vi "Enable Transient Operation.vi"(8 "error in (no error)":errorcluster, 10 "Enable Transient (T: Enable)":bool=TRUE, 11 "VISA resource name":refnum<visa-resource-name>) -> (0 "error out":errorcluster, 3 "VISA resource name out":refnum<visa-resource-name>)   [LabVIEW 2018, in "BK Precision 8600 Series.lvlib"]
doc: "Enable or disable the state of transient operation. Transient operation must be enabled first before sending a trigger to initiate the operation.\n\nRun this vi after configuring transient operation parameters using <b>Configure Transient Operation.vi</b>."
uses:
  <instrlib>/BK Precision 8600 Series/BK Precision 8600 Series.lvlib
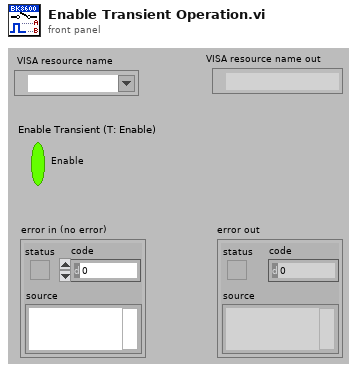
[diagram p1: front panel]
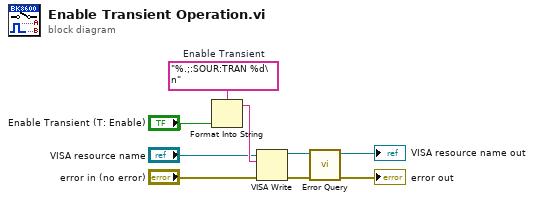
[diagram p0: block diagram]
diagram:
  w7 = "%.;:SOUR:TRAN %d\n"  # Enable Transient
  n1 = Format Into String(format string=w7, "Enable Transient (T: Enable)") -> (resulting string=w4:string)  [unwired: 2 in, 1 out]
  n2 = VISA Write(VISA resource name="VISA resource name", write buffer=w4, error in (no error)="error in (no error)") -> (VISA resource name out=w5:refnum<visa-resource-name>, error out=w6:errorcluster)  [unwired: 1 out]
  n3 = call <instrlib>:"Error Query.vi"("error in (no error)"=w6, "VISA resource name"=w5) -> ("error out"=→"error out":errorcluster, "VISA resource name out"=→"VISA resource name out":refnum<visa-resource-name>)  [unwired: 6 in, 2 out]
